vi "Ctor.vi"(8 "error in (no error)":errorcluster, 11 "ButtonControlEditorPanel in":refnum<class "ButtonControlEditorPanel.lvclass">) -> (0 "error out":errorcluster, 3 "ButtonControlEditorPanel out":refnum<class "ButtonControlEditorPanel.lvclass">)   [LabVIEW 2020, in "VolatusGUIControls.lvlib" / "ButtonControlEditorPanel.lvclass"]
uses:
  ButtonControlEditorPanel.lvclass
  ElementEditorPanel/ElementEditorPanel.lvclass
  ButtonControlEditorPanel.lvclass/ButtonControlEditorPanel.ctl
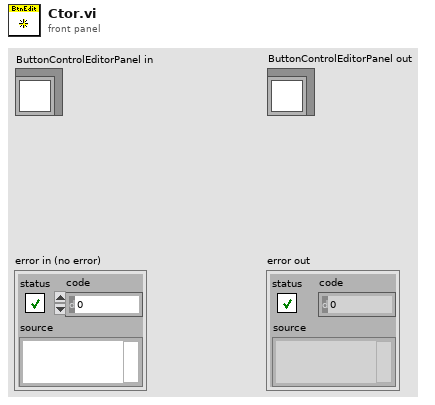
[diagram p1: front panel]
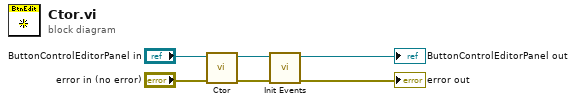
[diagram p0: block diagram]
diagram:
  n1 = call-parent "Ctor.vi"("error in (no error)"="error in (no error)", "ElementEditorPanel in"="ButtonControlEditorPanel in") -> ("error out"=w3:errorcluster, "ElementEditorPanel out"=w1:refnum<class "ButtonControlEditorPanel.lvclass">)  [unwired: 8 in]
  n2 = call "Init Events.vi"("error in (no error)"=w3, "ButtonControlEditorPanel in"=w1) -> ("error out"=→"error out":errorcluster, "ButtonControlEditorPanel out"=→"ButtonControlEditorPanel out":refnum<class "ButtonControlEditorPanel.lvclass">)  [unwired: 8 in]
